vi "DataSetValuesToDVR.vi"(8 "error in (no error)":errorcluster, 11 "dataset values":sgl[](array[numeric])) -> (0 "error out":errorcluster, 3 "new dataset values dvr":refnum<data-value>)   [LabVIEW 2017, in "DataEventCreator.lvlib"]
uses:
  <vilib>/addons/InsightCM/Devices/Shared/Common/DataEventCreator/DataEventCreator.lvlib
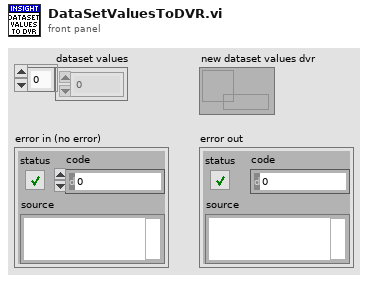
[diagram p1: front panel]
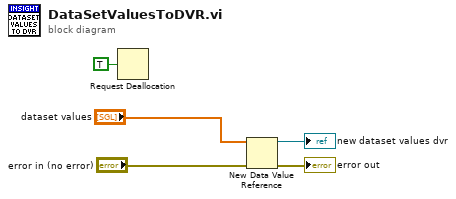
[diagram p0: block diagram]
diagram:
  n1 = Request Deallocation(TRUE ("flag")) -> ()
  n2 = New Data Value Reference(data value="dataset values", error in="error in (no error)") -> (data value reference=→"new dataset values dvr":refnum<data-value>, error out=→"error out":errorcluster)
